vi "OnDataDone Event Callback - ReadZ.vi"(4 "User Parameter":T1, 5 "Event Data":cluster{"Status":i32}, 6 "Control Ref":refnum<k7>, 7 "Event Common Data":T2) -> ()   [LabVIEW 2018]
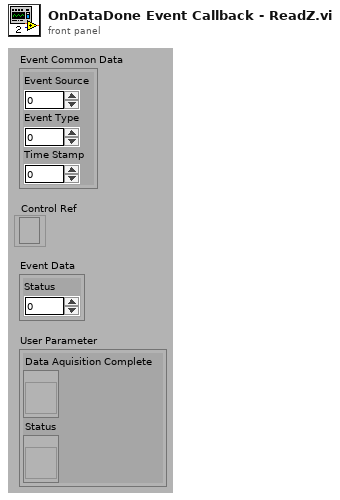
[diagram p1: front panel]
types:
  T1 = cluster{"Data Aquisition Complete":refnum<vi>, "Status":refnum<vi>}
  T2 = cluster{"Event Source":i32, "Event Type":u32, "Time Stamp":u32}
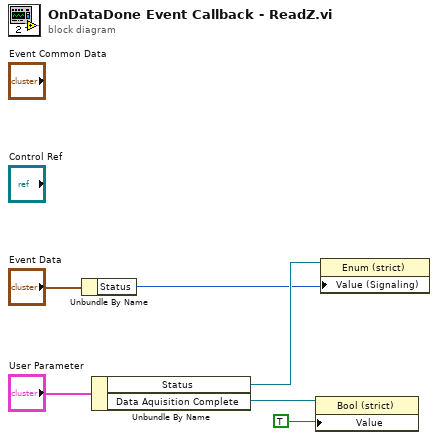
[diagram p0: block diagram]
diagram:
  n1 = Unbundle By Name("Event Data") -> ("Status"=w1:i32)
  n2 = Unbundle By Name("User Parameter") -> ("Status"=w3:refnum<vi>, "Data Aquisition Complete"=w5:refnum<vi>)
  n3 = property class="Bool (strict)"(reference=w5, "Value"=TRUE) -> ()  [unwired: 1 in, 2 out]
  n4 = property class="Enum (strict)"(reference=w3, "Value (Signaling)"=w1) -> ()  [unwired: 1 in, 2 out]
